vi "Main.vi"() -> ()   [LabVIEW 2011]
uses:
  GlobalVariables.vi
  <vilib>/lvdsc/process/internal/PRC_DeployLibraries.vi
  <vilib>/lvdsc/NI_DSC.lvlib
panel:
  out "Ready":bool
  in  "Open Schematic VI":bool
  in  "Open Ion Guage VI":bool
  in  "Open DeviceNet VI":bool
  in  "Open Vacuum Pump VI":bool
  in  "stop":bool
  in  "Open Festo VI":bool
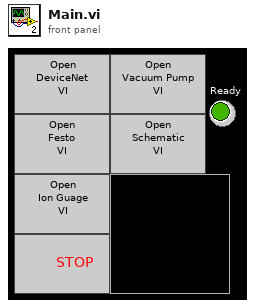
[diagram p1: front panel]
types:
  T1 = typedef "Device Cluster.ctl" = cluster{"Dnet":string, "Node":i32, "Type":string, "ID Number":u8, "SCCM":dbl, "FullScale":dbl, "Input Bytes":i32, "Output Bytes":i32, "Input Start Location":i32, "Output Start Location":i32, "Enabled":bool, "Bytes":u8[]}
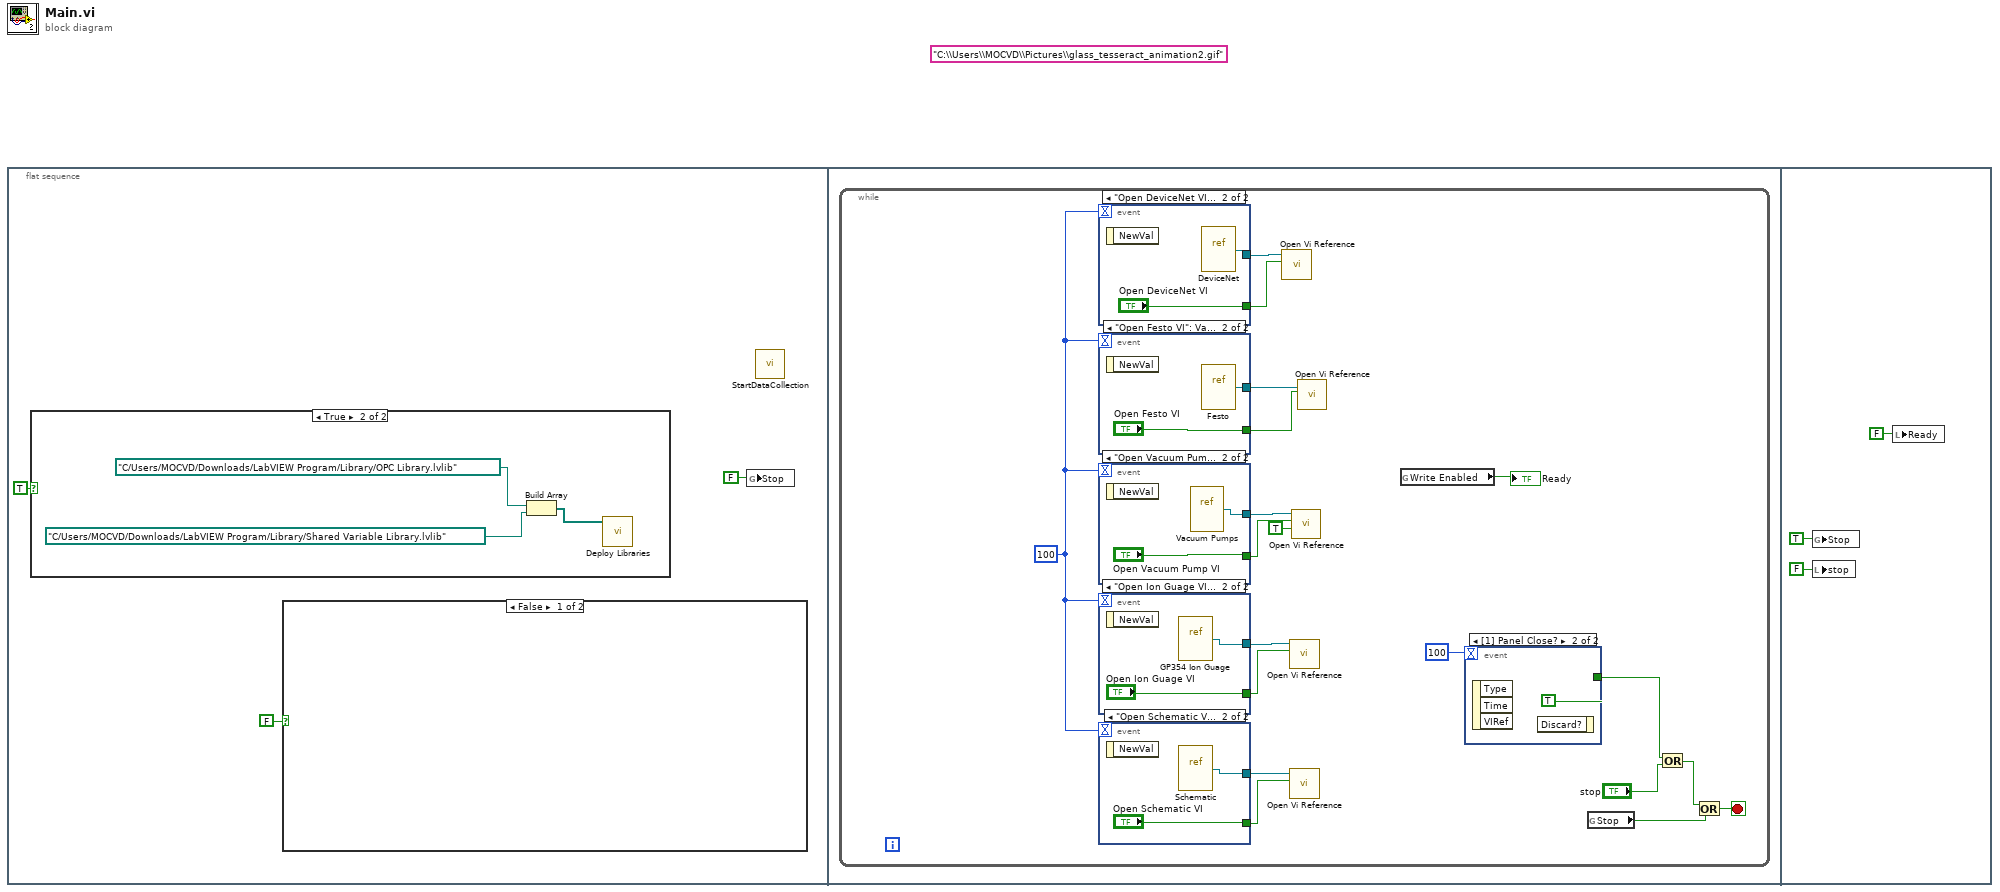
[diagram p0: block diagram]
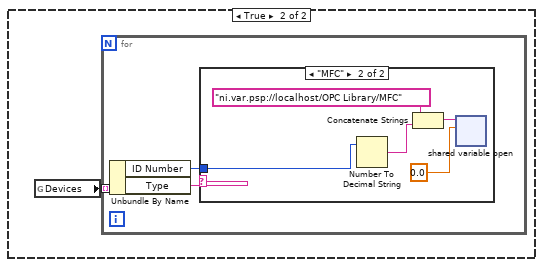
[diagram p3: hidden frame]
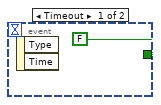
[diagram p5: hidden frame]
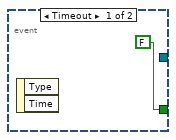
[diagram p6: hidden frame]
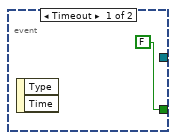
[diagram p7: hidden frame]
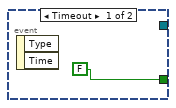
[diagram p8: hidden frame]
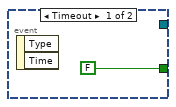
[diagram p9: hidden frame]
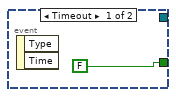
[diagram p10: hidden frame]
diagram:
  (unwired) "C:\\Users\\MOCVD\\Pictures\\glass_tesseract_animation2.gif" ("URL")
  n1 = flat-sequence {
    frame #0 {
      n2 = case shown="True" TRUE {
        frame False {
        }
        frame True {
          n3 = Build Array(path "C:/Users/MOCVD/Downloads/LabVIEW Program/Library/OPC Library.lvlib" ("library path"), path "C:/Users/MOCVD/Downloads/LabVIEW Program/Library/Shared Variable Library.lvlib" ("library path")) -> (w4:path[])
          n4 = call-poly <vilib>:"Deploy Libraries.vi"("library paths"=w4) -> ()  [unwired: 8 in, 1 out]
        }
      }
      n5 = case shown="False" FALSE {
        frame False {
        }
        frame True {
          n6 = global read "GlobalVariables.vi" "Devices"() -> (w7:T1[])
          n7 = for {
            tunnel: [w10] -> _ mode=indexing
            tunnel: w7 -> [w10] mode=indexing
            n8 = Unbundle By Name(w10) -> ("ID Number"=w8:u8, "Type"=w9:string)
            n9 = case shown="\"MFC\"" w9 {
              tunnel: w8 -> [_ w14]
              frame Default {
              }
              frame "MFC" {
                n10 = Number To Decimal String(number=w14) -> (decimal integer string=w15:string)  [unwired: 1 in]
                n11 = Concatenate Strings("ni.var.psp://localhost/OPC Library/MFC", w15) -> (w12:string)
                n12 = shared-variable-open(w12, 0.0) -> ()  [unwired: 3 in, 2 out]
              }
            }
          }
        }
      }
      n13 = global write "GlobalVariables.vi" "Stop"(FALSE ("Stop")) -> ()
      n14 = call "StartDataCollection.vi"() -> ()  [unwired: 12 in]
    }
    frame #1 {
      n15 = while {
        stop <- w33 stop-if-true
        w22 = 100
        n16 = event shown="[1] \"Open DeviceNet VI\": Value Change" {
          selector: _ -> [_ _]
          dyn-events: _ -> [_ _]
          timeout: w22 -> [_ _]
          tunnel: [FALSE ("Open DeviceNet VI") "Open DeviceNet VI"] -> w25
          tunnel: [_ w44] -> w26
          event Timeout {
            n17 = event-data() -> ()  [unwired: 1 in, 2 out]
          }
          event "Open DeviceNet VI": Value Change {
            n18 = event-data() -> ()  [unwired: 1 in, 1 out]
            n19 = vi-ref "DeviceNet.vi"() -> (w44:refnum<vi>)
          }
        }
        n20 = event shown="[1] \"Open Festo VI\": Value Change" {
          selector: _ -> [_ _]
          dyn-events: _ -> [_ _]
          timeout: w22 -> [_ _]
          tunnel: [FALSE ("Open Festo VI") "Open Festo VI"] -> w27
          tunnel: [_ w50] -> w28
          event Timeout {
            n21 = event-data() -> ()  [unwired: 1 in, 2 out]
          }
          event "Open Festo VI": Value Change {
            n22 = event-data() -> ()  [unwired: 1 in, 1 out]
            n23 = vi-ref "Festo.vi"() -> (w50:refnum<vi>)
          }
        }
        n24 = event shown="[1] \"Open Vacuum Pump VI\": Value Change" {
          selector: _ -> [_ _]
          dyn-events: _ -> [_ _]
          timeout: w22 -> [_ _]
          tunnel: [FALSE ("Open Vacuum Pump VI") "Open Vacuum Pump VI"] -> w31
          tunnel: [_ w47] -> w32
          event Timeout {
            n25 = event-data() -> ()  [unwired: 1 in, 2 out]
          }
          event "Open Vacuum Pump VI": Value Change {
            n26 = event-data() -> ()  [unwired: 1 in, 1 out]
            n27 = vi-ref "Vacuum Pumps.vi"() -> (w47:refnum<vi>)
          }
        }
        n28 = event shown="[1] \"Open Ion Guage VI\": Value Change" {
          selector: _ -> [_ _]
          dyn-events: _ -> [_ _]
          timeout: w22 -> [_ _]
          tunnel: [FALSE ("Open Festo VI") "Open Ion Guage VI"] -> w29
          tunnel: [_ w41] -> w30
          event Timeout {
            n29 = event-data() -> ()  [unwired: 1 in, 2 out]
          }
          event "Open Ion Guage VI": Value Change {
            n30 = event-data() -> ()  [unwired: 1 in, 1 out]
            n31 = vi-ref "GP354 Ion Guage.vi"() -> (w41:refnum<vi>)
          }
        }
        n32 = event shown="[1] \"Open Schematic VI\": Value Change" {
          selector: _ -> [_ _]
          dyn-events: _ -> [_ _]
          timeout: w22 -> [_ _]
          tunnel: [FALSE ("Open Festo VI") "Open Schematic VI"] -> w23
          tunnel: [_ w39] -> w24
          event Timeout {
            n33 = event-data() -> ()  [unwired: 1 in, 2 out]
          }
          event "Open Schematic VI": Value Change {
            n34 = event-data() -> ()  [unwired: 1 in, 1 out]
            n35 = vi-ref "Schematic.vi"() -> (w39:refnum<vi>)
          }
        }
        n36 = call "Open Vi Reference.vi"("RunVi"=w25, "reference"=w26) -> ()  [unwired: 2 in, 2 out]
        n37 = call "Open Vi Reference.vi"("RunVi"=w29, "reference"=w30) -> ()  [unwired: 2 in, 2 out]
        n38 = call "Open Vi Reference.vi"("RunVi"=w23, "reference"=w24) -> ()  [unwired: 2 in, 2 out]
        n39 = call "Open Vi Reference.vi"("Show"=TRUE, "RunVi"=w31, "reference"=w32) -> ()  [unwired: 1 in, 2 out]
        n40 = call "Open Vi Reference.vi"("RunVi"=w27, "reference"=w28) -> ()  [unwired: 2 in, 2 out]
        n41 = global read "GlobalVariables.vi" "Write Enabled"() -> (→"Ready":bool)
        n42 = event shown="[1] Panel Close?" {
          selector: _ -> [_ _]
          dyn-events: _ -> [_ _]
          timeout: 100 -> [_ _]
          tunnel: [FALSE ("y") TRUE ("y")] -> w17
          event Timeout {
            n43 = event-data() -> ()  [unwired: 1 in, 2 out]
          }
          event Panel Close? {
            n44 = event-data() -> ()  [unwired: 1 in, 3 out]
            n45 = event-data() -> ()  [unwired: 2 in, 1 out]
          }
        }
        n46 = global read "GlobalVariables.vi" "Stop"() -> (w34:bool)
        n47 = Or(x=w17, y="stop") -> (x .or. y?=w19:bool)
        n48 = Or(x=w19, y=w34) -> (x .or. y?=w33:bool)
      }
    }
    frame #2 {
      n49 = global write "GlobalVariables.vi" "Stop"(TRUE ("Stop")) -> ()
      n50 = local write "stop"(FALSE ("stop")) -> ()
      n51 = local write "Ready"(FALSE ("Ready")) -> ()
    }
  }
